vi "Reset FPGA.vi"(8 "Error In":errorcluster) -> (0 "error out":errorcluster)   [LabVIEW 2017, in "Logger.lvclass"]
uses:
  Logger.lvclass
  <vilib>/FPGAPlugInAG/Dynamic/niLvFpga_Reset_Dynamic.vi
  <vilib>/FPGAPlugInAG/Dynamic/niLvFpga_Close_Dynamic.vi
  <vilib>/rvi/interface/nirviMethod/nirviMethod.xnode
  <vilib>/rvi/interface/nirviCloseFPGA/nirviCloseFPGA.xnode
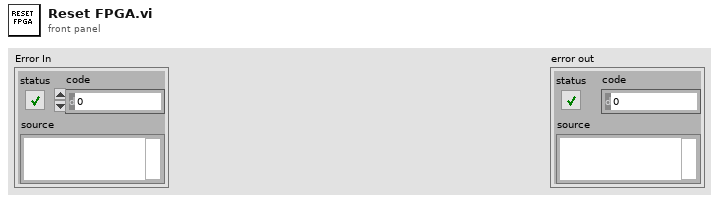
[diagram p1: front panel]
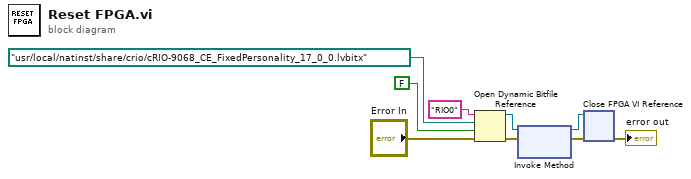
[diagram p0: block diagram]
diagram:
  n1 = Open Dynamic Bitfile Reference(0:"RIO0" ("Device address"), 1:path "/usr/local/natinst/share/crio/cRIO-9068_CE_FixedPersonality_17_0_0.lvbitx" ("Bitfile path"), 2:FALSE ("Run When Loaded"), 3:"Error In") -> (5:w9:refnum<k20>, 8:w8:errorcluster)  [unwired: 1 in]
  n2 = xnode "Invoke Method"("FPGA VI Reference In"=w9, "error in"=w8) -> ("FPGA VI Reference Out"=w7:refnum<k20>, "error out"=w6:errorcluster)
  n3 = xnode "Close FPGA VI Reference"("FPGA VI Reference In"=w7, "error in"=w6) -> ("error out"=→"error out":errorcluster)
